vi "Update control status.vi"(8 "error in (no error)":errorcluster caption="entrée d'erreur (pas d'erreur)", 10 "Control-Client old":refnum<class "Control-Client.lvclass">, 11 "Control-Client new":refnum<class "Control-Client.lvclass">) -> (0 "error out":errorcluster caption="sortie d'erreur", 3 "Control-Client en sortie":refnum<class "Control-Client.lvclass">)   [LabVIEW 2015, in "Control-Client.lvclass"]
uses:
  Control-Client.lvclass
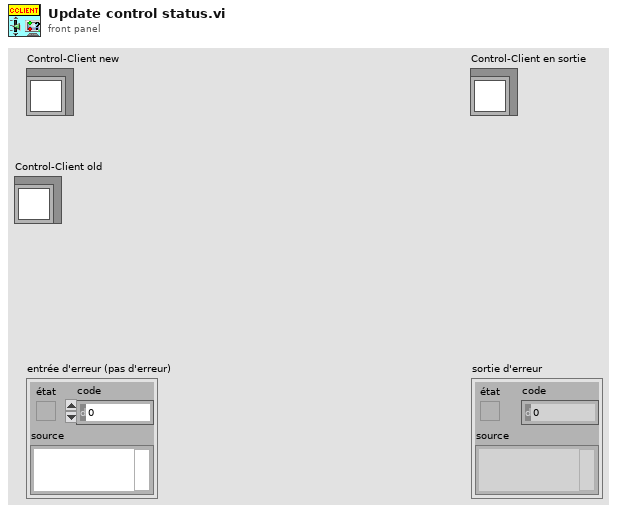
[diagram p1: front panel]
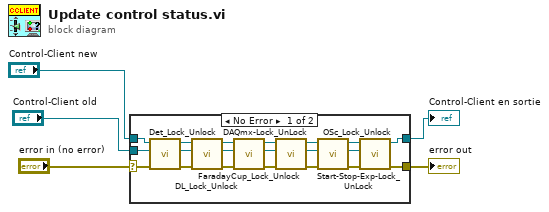
[diagram p0: block diagram]
diagram:
  n1 = case shown="No Error" "error in (no error)" {
    selector: "error in (no error)" -> [w15 w26]
    tunnel: [w8 w27] -> w3
    tunnel: "Control-Client new" -> [w24 w27]
    tunnel: "Control-Client old" -> [w25 _]
    tunnel: [w6 w26] -> w1
    frame No Error {
      n2 = call "Det_Lock_Unlock.vi"("entrée d'erreur (pas d'erreur)"=w15, "Control-Client old entrée"=w25, "Control-Client new entrée"=w24) -> ("sortie d'erreur"=w21:errorcluster, "Control-Client old out"=w22:refnum<class "Control-Client.lvclass">, "Control-Client new out"=w23:refnum<class "Control-Client.lvclass">)  [unwired: 6 in]
      n3 = call "DL_Lock_Unlock.vi"("entrée d'erreur (pas d'erreur)"=w21, "Control-Client old entrée"=w22, "Control-Client new entrée"=w23) -> ("sortie d'erreur"=w16:errorcluster, "Control-Client old out"=w19:refnum<class "Control-Client.lvclass">, "Control-Client new out"=w20:refnum<class "Control-Client.lvclass">)  [unwired: 6 in]
      n4 = call "FaradayCup_Lock_Unlock.vi"("entrée d'erreur (pas d'erreur)"=w16, "Control-Client old entrée"=w19, "Control-Client new entrée"=w20) -> ("sortie d'erreur"=w14:errorcluster, "Control-Client old out"=w17:refnum<class "Control-Client.lvclass">, "Control-Client new out"=w18:refnum<class "Control-Client.lvclass">)  [unwired: 6 in]
      n5 = call "DAQmx-Lock_UnLock.vi"("entrée d'erreur (pas d'erreur)"=w14, "Control-Client old entrée"=w17, "Control-Client new entrée"=w18) -> ("sortie d'erreur"=w11:errorcluster, "Control-Client old out"=w12:refnum<class "Control-Client.lvclass">, "Control-Client new out"=w13:refnum<class "Control-Client.lvclass">)  [unwired: 6 in]
      n6 = call "Start-Stop-Exp-Lock_UnLock.vi"("entrée d'erreur (pas d'erreur)"=w11, "Control-Client old entrée"=w12, "Control-Client new entrée"=w13) -> ("sortie d'erreur"=w7:errorcluster, "Control-Client old out"=w9:refnum<class "Control-Client.lvclass">, "Control-Client new out"=w10:refnum<class "Control-Client.lvclass">)  [unwired: 6 in]
      n7 = call "OSc_Lock_Unlock.vi"("entrée d'erreur (pas d'erreur)"=w7, "Control-Client old entrée"=w9, "Control-Client new entrée"=w10) -> ("sortie d'erreur"=w6:errorcluster, "Control-Client new out"=w8:refnum<class "Control-Client.lvclass">)  [unwired: 6 in, 1 out]
    }
    frame Error {
    }
  }
  "error out" <- w1
  "Control-Client en sortie" <- w3
